vi "main_serial_communication.vi"() -> ()   [LabVIEW 2015]
panel:
  out "Center 2":sgl(graph)
  in  "MFC 3":bool
  in  "MFC 2":bool
  in  "MFC 1":bool
  in  "Delay(ms)":u32
  out "호퍼2":sgl(graph)
  out "호퍼1":sgl(graph)
  in  "?":bool
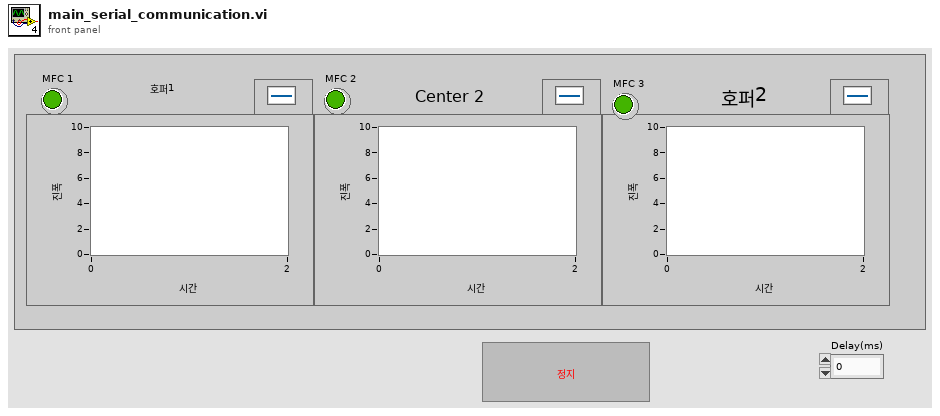
[diagram p1: front panel]
types:
  T1 = typedef "MFC_Address.ctl" = string
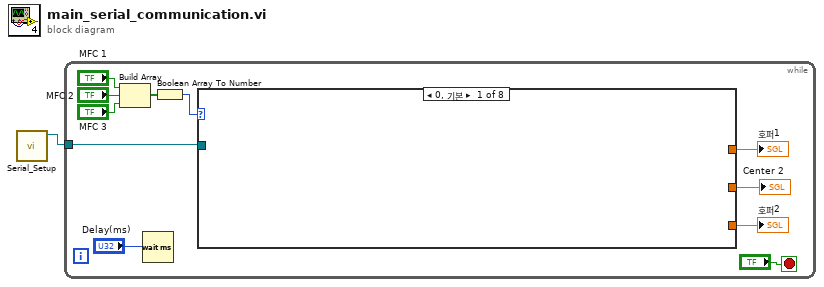
[diagram p0: block diagram]
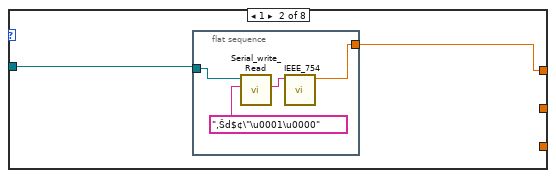
[diagram p2: hidden frame]
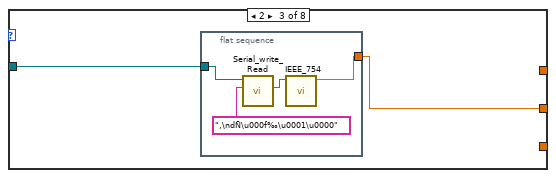
[diagram p3: hidden frame]
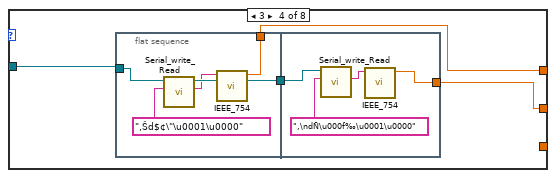
[diagram p4: hidden frame]
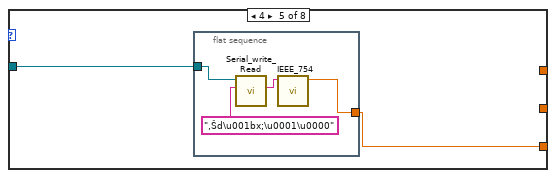
[diagram p5: hidden frame]
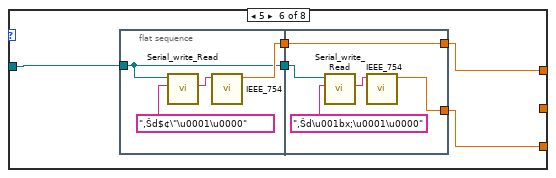
[diagram p6: hidden frame]
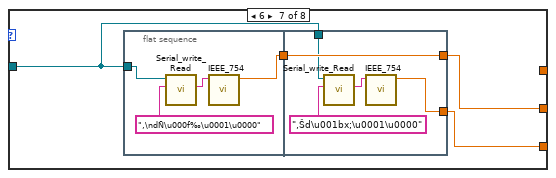
[diagram p7: hidden frame]
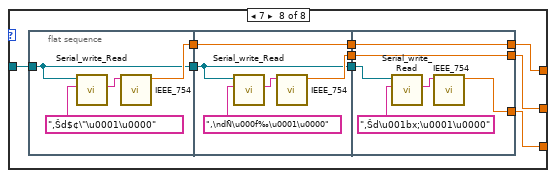
[diagram p8: hidden frame]
diagram:
  n1 = call "Serial_Setup.vi"() -> ("VISA resource name out"=w1:refnum<visa-resource-name>)  [unwired: 10 in, 1 out]
  n2 = while {
    tunnel: w1 -> [w8]
    stop <- "?" stop-if-true
    n3 = Build Array("MFC 1", "MFC 2", "MFC 3") -> (w5:bool[])
    n4 = Wait (ms)(milliseconds to wait="Delay(ms)") -> ()  [unwired: 1 out]
    n5 = Boolean Array To Number(Boolean array=w5) -> (number=w4:u32)
    n6 = case shown="0, 기본" w4 {
      tunnel: w8 -> [_ w14 w20 w28 w39 w47 w58 w73]
      tunnel: [_ w13 _ w26 _ w45 _ w77] -> w10
      tunnel: [_ _ _ _ w38 w44 w59 w74] -> w9
      tunnel: [_ _ w19 w25 _ _ w60 w75] -> w3
      frame 0, Default {
      }
      frame 1 {
        n7 = flat-sequence {
          tunnel: w14 -> [w15]
          tunnel: [w16] -> w13
          frame #0 {
            n8 = call "Serial_write_Read.vi"("Command"="‚Šd$¢\"\u0001\u0000", "VISA 리소스 이름"=w15) -> ("Response"=w17:T1)  [unwired: 6 in, 3 out]
            n9 = call "IEEE_754.vi"("input"=w17) -> ("Return"=w16:sgl)  [unwired: 10 in]
          }
        }
      }
      frame 2 {
        n10 = flat-sequence {
          tunnel: [w22] -> w19
          tunnel: w20 -> [w21]
          frame #0 {
            n11 = call "Serial_write_Read.vi"("Command"="‚\ndÑ\u000f‰\u0001\u0000", "VISA 리소스 이름"=w21) -> ("Response"=w24:T1)  [unwired: 6 in, 3 out]
            n12 = call "IEEE_754.vi"("input"=w24) -> ("Return"=w22:sgl)  [unwired: 10 in]
          }
        }
      }
      frame 3 {
        n13 = flat-sequence {
          tunnel: w28 -> [w32]
          tunnel: [w31] -> w27
          tunnel: [w29] -> w26
          tunnel: w27 -> [w36]
          tunnel: [w34] -> w25
          frame #0 {
            n14 = call "Serial_write_Read.vi"("Command"="‚Šd$¢\"\u0001\u0000", "VISA 리소스 이름"=w32) -> ("Response"=w30:T1, "VISA 리소스 이름 출력"=w31:refnum<visa-resource-name>)  [unwired: 6 in, 2 out]
            n15 = call "IEEE_754.vi"("input"=w30) -> ("Return"=w29:sgl)  [unwired: 10 in]
          }
          frame #1 {
            n16 = call "Serial_write_Read.vi"("Command"="‚\ndÑ\u000f‰\u0001\u0000", "VISA 리소스 이름"=w36) -> ("Response"=w35:T1)  [unwired: 6 in, 3 out]
            n17 = call "IEEE_754.vi"("input"=w35) -> ("Return"=w34:sgl)  [unwired: 10 in]
          }
        }
      }
      frame 4 {
        n18 = flat-sequence {
          tunnel: [w41] -> w38
          tunnel: w39 -> [w40]
          frame #0 {
            n19 = call "Serial_write_Read.vi"("Command"="‚Šd\u001bx;\u0001\u0000", "VISA 리소스 이름"=w40) -> ("Response"=w42:T1)  [unwired: 6 in, 3 out]
            n20 = call "IEEE_754.vi"("input"=w42) -> ("Return"=w41:sgl)  [unwired: 10 in]
          }
        }
      }
      frame 5 {
        n21 = flat-sequence {
          tunnel: [w50] -> w48
          tunnel: w47 -> [w49]
          tunnel: [w49] -> w46
          tunnel: w48 -> [w57]
          tunnel: [w57] -> w45
          tunnel: [w54] -> w44
          tunnel: w46 -> [w53]
          frame #0 {
            n22 = call "Serial_write_Read.vi"("Command"="‚Šd$¢\"\u0001\u0000", "VISA 리소스 이름"=w49) -> ("Response"=w51:T1)  [unwired: 6 in, 3 out]
            n23 = call "IEEE_754.vi"("input"=w51) -> ("Return"=w50:sgl)  [unwired: 10 in]
          }
          frame #1 {
            n24 = call "Serial_write_Read.vi"("Command"="‚Šd\u001bx;\u0001\u0000", "VISA 리소스 이름"=w53) -> ("Response"=w55:T1)  [unwired: 6 in, 3 out]
            n25 = call "IEEE_754.vi"("input"=w55) -> ("Return"=w54:sgl)  [unwired: 10 in]
          }
        }
      }
      frame 6 {
        n26 = flat-sequence {
          tunnel: [w63] -> w61
          tunnel: w58 -> [w62]
          tunnel: w61 -> [w70]
          tunnel: [w70] -> w60
          tunnel: [w67] -> w59
          tunnel: w58 -> [w66]
          frame #0 {
            n27 = call "Serial_write_Read.vi"("Command"="‚\ndÑ\u000f‰\u0001\u0000", "VISA 리소스 이름"=w62) -> ("Response"=w65:T1)  [unwired: 6 in, 3 out]
            n28 = call "IEEE_754.vi"("input"=w65) -> ("Return"=w63:sgl)  [unwired: 10 in]
          }
          frame #1 {
            n29 = call "Serial_write_Read.vi"("Command"="‚Šd\u001bx;\u0001\u0000", "VISA 리소스 이름"=w66) -> ("Response"=w68:T1)  [unwired: 6 in, 3 out]
            n30 = call "IEEE_754.vi"("input"=w68) -> ("Return"=w67:sgl)  [unwired: 10 in]
          }
        }
      }
      frame 7 {
        n31 = flat-sequence {
          tunnel: [w81] -> w79
          tunnel: w73 -> [w80]
          tunnel: [w80] -> w72
          tunnel: w79 -> [w88]
          tunnel: [w88] -> w78
          tunnel: [w85] -> w76
          tunnel: w72 -> [w84]
          tunnel: [w84] -> w71
          tunnel: w78 -> [w94]
          tunnel: [w94] -> w77
          tunnel: w76 -> [w93]
          tunnel: [w93] -> w75
          tunnel: [w90] -> w74
          tunnel: w71 -> [w89]
          frame #0 {
            n32 = call "Serial_write_Read.vi"("Command"="‚Šd$¢\"\u0001\u0000", "VISA 리소스 이름"=w80) -> ("Response"=w82:T1)  [unwired: 6 in, 3 out]
            n33 = call "IEEE_754.vi"("input"=w82) -> ("Return"=w81:sgl)  [unwired: 10 in]
          }
          frame #1 {
            n34 = call "Serial_write_Read.vi"("Command"="‚\ndÑ\u000f‰\u0001\u0000", "VISA 리소스 이름"=w84) -> ("Response"=w87:T1)  [unwired: 6 in, 3 out]
            n35 = call "IEEE_754.vi"("input"=w87) -> ("Return"=w85:sgl)  [unwired: 10 in]
          }
          frame #2 {
            n36 = call "Serial_write_Read.vi"("Command"="‚Šd\u001bx;\u0001\u0000", "VISA 리소스 이름"=w89) -> ("Response"=w91:T1)  [unwired: 6 in, 3 out]
            n37 = call "IEEE_754.vi"("input"=w91) -> ("Return"=w90:sgl)  [unwired: 10 in]
          }
        }
      }
    }
    "호퍼1" <- w10
    "호퍼2" <- w9
    "Center 2" <- w3
  }
